vi "ModifyGraph height.vi"(8 "error in (no error)":errorcluster, 10 "height (points) [256]":dbl=256.0, 11 "ITX Commands in":refnum<class "ITX Commands.lvclass">) -> (0 "error out":errorcluster, 3 "ITX Commands out":refnum<class "ITX Commands.lvclass">)   [LabVIEW 2019, in "ITX Commands.lvclass"]
uses:
  ITX Commands.lvclass
panel:
  out "resulting string":string
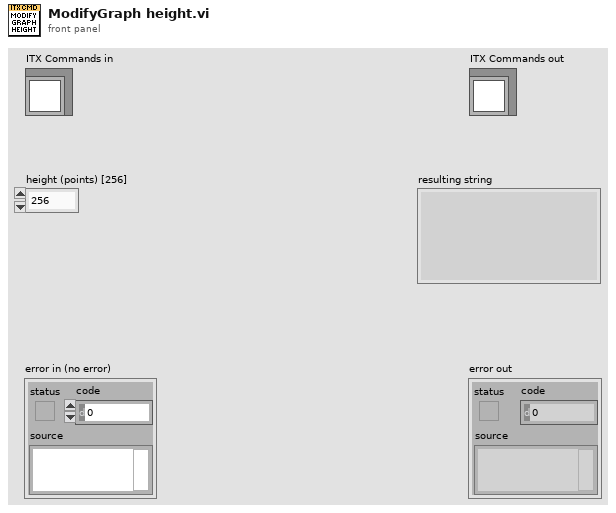
[diagram p1: front panel]
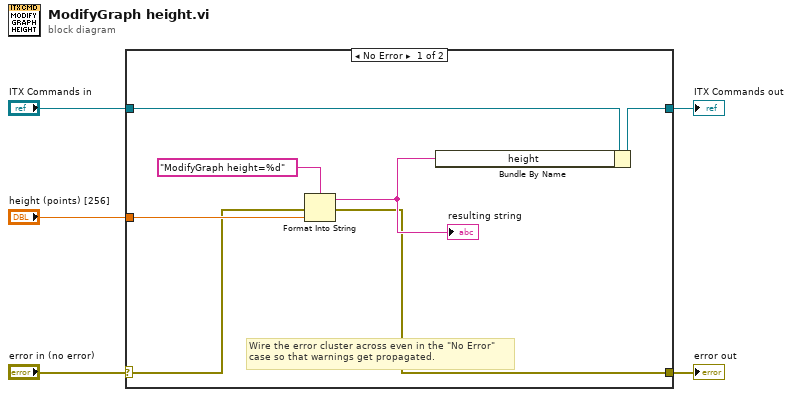
[diagram p0: block diagram]
diagram:
  n1 = case shown="No Error" "error in (no error)" {
    selector: "error in (no error)" -> [w7 w14]
    tunnel: [w6 w14] -> w4
    tunnel: [w9 w13] -> w2
    tunnel: "ITX Commands in" -> [w10 w13]
    tunnel: "height (points) [256]" -> [w8 _]
    frame No Error {
      # "Wire the error cluster across even in the \"No Error\"\ncase so that warnings get propagated."
      n2 = Format Into String(format string="ModifyGraph height=%d", error in=w7, w8) -> (resulting string=w11:string, error out=w6:errorcluster)  [unwired: 1 in]
      "resulting string" <- w11
      n3 = Bundle By Name(cluster=w10, "height"=w11) -> (w9:refnum<class "ITX Commands.lvclass">)
    }
    frame Error {
    }
  }
  "error out" <- w4
  "ITX Commands out" <- w2
